vi "ReleaseMutex.vi"(4 "error in (no error)":errorcluster, 6 "CloseHandle? (f)":bool, 7 "hMutex (NULL)":i32 format="%.0x") -> (0 "error out":errorcluster)   [LabVIEW 2011]
uses:
  KERNEL32.DLL
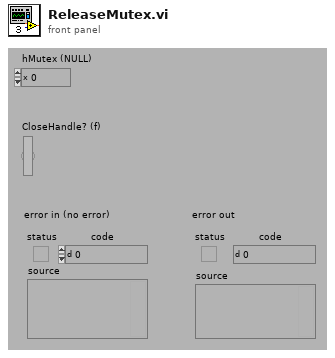
[diagram p1: front panel]
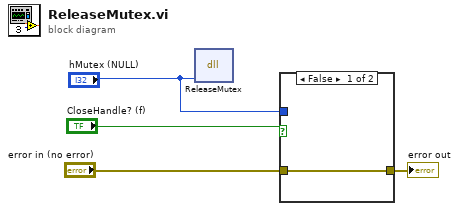
[diagram p0: block diagram]
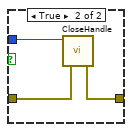
[diagram p2: hidden frame]
diagram:
  n1 = dll-call lib="KERNEL32.DLL" fn="ReleaseMutex" label="ReleaseMutex()"("hMutex"="hMutex (NULL)") -> ()  [unwired: 4 in, 3 out]
  n2 = case shown="False" "CloseHandle? (f)" {
    tunnel: "error in (no error)" -> [w5 w8]
    tunnel: [w5 w7] -> w3
    tunnel: "hMutex (NULL)" -> [_ w6]
    frame False {
    }
    frame True {
      n3 = call "CloseHandle.vi"("error in (no error)"=w8, "hObject (NULL)"=w6) -> ("error out"=w7:errorcluster)  [unwired: 5 out]
    }
  }
  "error out" <- w3
